vi "Read Step UI Main VI Ref.vi"(8 "error in (no error)":errorcluster, 11 "Wait Step UI in":refnum<class "Wait Step UI.lvclass">) -> (0 "error out":errorcluster, 2 "Step UI Main VI Ref":refnum<vi>, 3 "Wait Step UI out":refnum<class "Wait Step UI.lvclass">)   [LabVIEW 2015, in "Wait Step UI.lvclass"]
uses:
  Wait Step UI.lvclass
  Step UI Main.vi
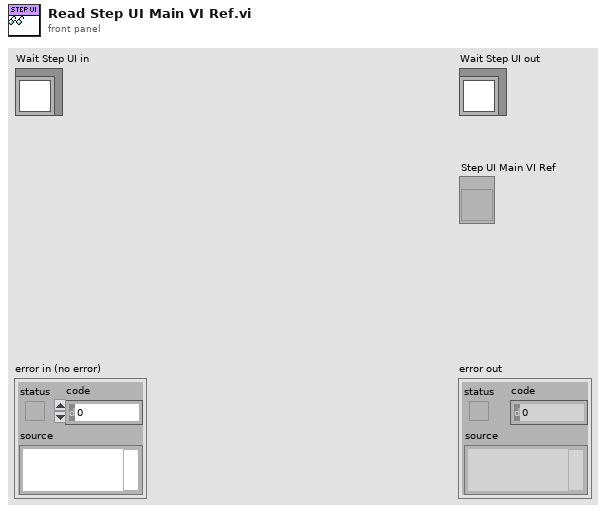
[diagram p1: front panel]
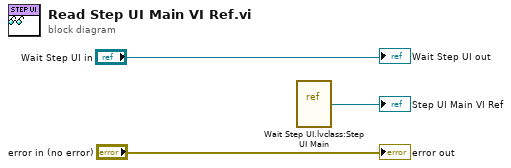
[diagram p0: block diagram]
diagram:
  n1 = vi-ref "Wait Step UI.lvclass:Step UI Main.vi"() -> (→"Step UI Main VI Ref":refnum<vi>)
  "error out" <- "error in (no error)"
  "Wait Step UI out" <- "Wait Step UI in"
